vi "Control Lift.vi"(0 "Loop Time (ms)":u32=10, 2 "Lift Min Speed to Raise at (%)":dbl=-0.35, 5 "Lift Up PID Terms":cluster{"Kp":dbl, "Ki":dbl, "Kd":dbl}={"Kp"=0.1, "Ki"=0.0, "Kd"=0.0}) -> (14 "PID Tracking Lift Up":T1(graph)={"Goal"=0.0, "Process Variable"=-0.0345825, "Max Ouput"=0.0034582500000000004, 0.0345825, 0.0034582500000000004, 0.0, -0.0}, 15 "Current Error Lift":dbl=0.0345825)   [LabVIEW 2017]
uses:
  <vilib>/Rock Robotics/WPI/ThirdParty/Phoenix-LabVIEW/Motor Controller/Controls/CTRE_Phoenix_MotorControl_ControlMode.ctl
  <vilib>/Rock Robotics/WPI/DriverStation/WPI_DriverStationRobotMode2.ctl
  Globals/Robot Global Data.vi
  Globals/Manipulator Controller Inputs.vi
panel:
  in  "Lift Down Fast":bool=TRUE
  in  "Testing":bool
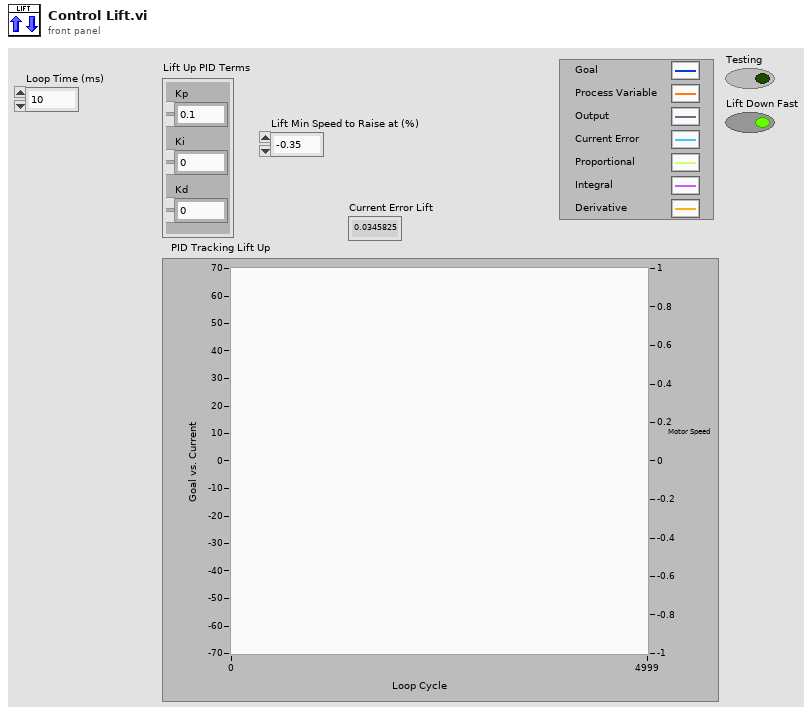
[diagram p1: front panel]
types:
  T1 = cluster{"Goal":dbl, "Process Variable":dbl, "Max Ouput":dbl, dbl, dbl, dbl, dbl}
  T2 = typedef "WPI_DriverStationRobotMode2.ctl" = enum16{"Autonomous Disabled", "Autonomous Enabled", "Teleop Disabled", "Teleop Enabled", "Disconnected", "Finish", "Test Disabled", "Test Enabled", "Emergency Stopped"}
  T3 = typedef "WPI_MotorControlDeviceRef.ctl" = cluster{"DeviceStatus":errorcluster, "Type":T4, "PWM":cluster{"PWM Channel":T5, "DeadBand":T6}, "CAN":cluster{"Device Number":u8, "SetOutput VI Ref":variant, "GetOutput VI Ref":variant, "Enable VI Ref":variant, "Disable VI Ref":variant, "Data":variant}, "Invert":bool, "DIO PWM":cluster{"PWM \"Enable\" Channel":T5, "DIOChannel":T7, "PWM Rate":dbl}}
  T4 = typedef "WPI_MotorControlType.ctl" = enum16{"PWM", "CAN", "DIO PWM"}
  T5 = typedef "FPGA_DIOPWMChannel.ctl" = enum8{"PWM 0", "PWM 1", "PWM 2", "PWM 3", "PWM 4", "PWM 5", "PWM 6", "PWM 7", "PWM 8", "PWM 9", "PWM MXP 0", "PWM MXP 1", "PWM MXP 2", "PWM MXP 3", "PWM MXP 4", "PWM MXP 5", "PWM MXP 6", "PWM MXP 7", "PWM MXP 8", "PWM MXP 9", "Invalid"}
  T6 = typedef "WPI_PWMDeadband.ctl" = cluster{"Name":string, "maxPositivePwm":i32, "minPositivePwm":i32, "centerPwm":i32, "maxNegativePwm":i32, "minNegativePwm":i32, "angularRange":u16}
  T7 = typedef "FPGA_DIOChannel.ctl" = enum8{"DIO 0", "DIO 1", "DIO 2", "DIO 3", "DIO 4", "DIO 5", "DIO 6", "DIO 7", "DIO 8", "DIO 9", "DIO MXP 0", "DIO MXP 1", "DIO MXP 2", "DIO MXP 3", "DIO MXP 4", "DIO MXP 5", "DIO MXP 6", "DIO MXP 7", "DIO MXP 8", "DIO MXP 9", "DIO MXP 10", "DIO MXP 11", "DIO MXP 12", "DIO MXP 13", "DIO MXP 14", "DIO MXP 15", "SPI Port CS1", "SPI Port CS2", "SPI Port CS3", "SPI Port MISO", "SPI Port MOSI", "Invalid"}
  T8 = typedef "CTRE_Phoenix_MotorControl_ControlMode.ctl" = u16
  T9 = typedef "WPI_DriverStationMatch Info.ctl" = cluster{"Autonomous Elapsed Seconds":dbl, "TeleOp Elapsed Seconds":dbl, "Disabled Elapsed Seconds":dbl, "Visited Autonomous":bool, "Visited TeleOp":bool, "Visited Disabled":bool, "Autonomous Settings":cluster{"Autonomous Style":enum16{"Iterative", "Independent"}, "VI Refnum":refnum<vi>}}
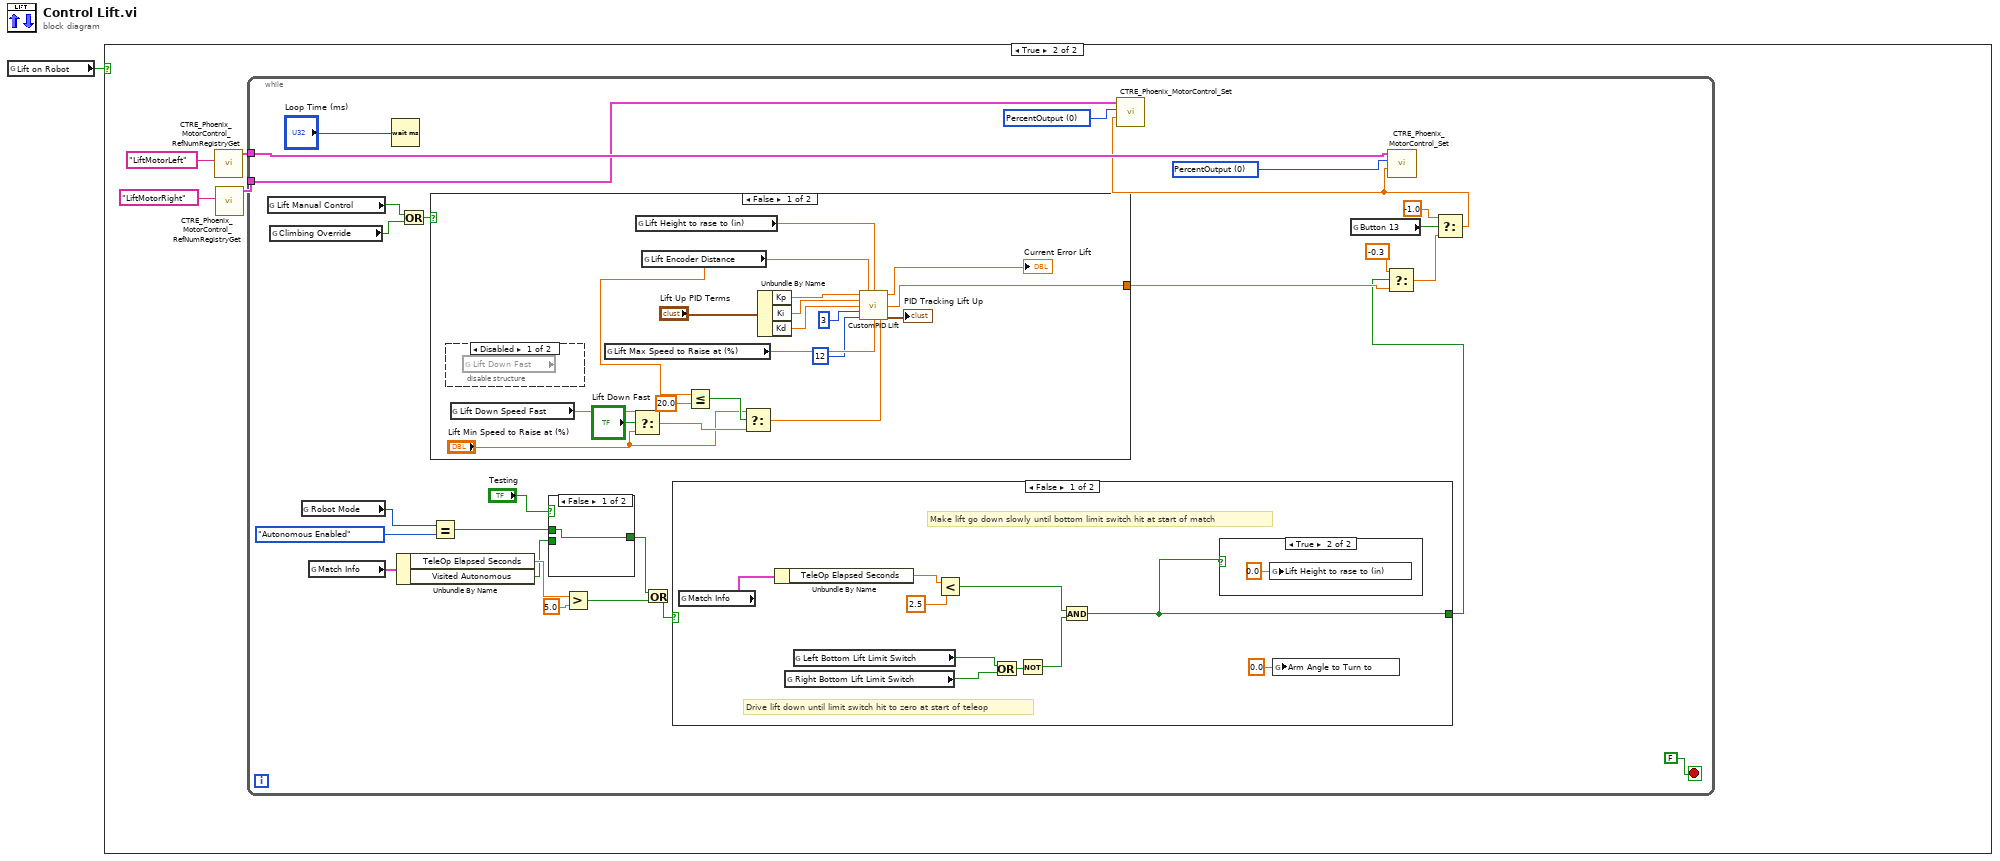
[diagram p0: block diagram]
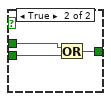
[diagram p3: hidden frame]
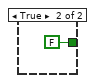
[diagram p5: hidden frame]
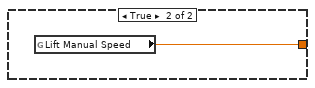
[diagram p7: hidden frame]
diagram:
  n1 = global read "Robot Global Data.vi" "Lift on Robot"() -> (w1:bool)
  n2 = case shown="True" w1 {
    frame False {
    }
    frame True {
      n3 = call "CTRE_Phoenix_MotorControl_RefNumRegistryGet.vi"("refnum name"="LiftMotorLeft") -> ("PhoenixMotorControlDevRef"=w5:T3)  [unwired: 9 in, 1 out]
      n4 = call "CTRE_Phoenix_MotorControl_RefNumRegistryGet.vi"("refnum name"="LiftMotorRight") -> ("PhoenixMotorControlDevRef"=w2:T3)  [unwired: 9 in, 1 out]
      n5 = while {
        tunnel: w5 -> [w31]
        tunnel: w2 -> [w27]
        stop <- FALSE stop-if-true
        w28 = T8 0 items=["PercentOutput"=0, "Position"=1, "Velocity"=2, "Current"=3, "Follower"=5, "MotionProfile"=6, "MotionMagic"=7, "MotionMagicArc"=8, "MotionProfileArc"=10, "Disabled"=15] ("Control Mode")
        w30 = T8 0 items=["PercentOutput"=0, "Position"=1, "Velocity"=2, "Current"=3, "Follower"=5, "MotionProfile"=6, "MotionMagic"=7, "MotionMagicArc"=8, "MotionProfileArc"=10, "Disabled"=15] ("Control Mode")
        n6 = global read "Robot Global Data.vi" "Lift Manual Control"() -> (w20:bool)
        n7 = global read "Robot Global Data.vi" "Climbing Override"() -> (w19:bool)
        n8 = global read "Robot Global Data.vi" "Robot Mode"() -> (w22:T2)
        n9 = global read "Robot Global Data.vi" "Match Info"() -> (w18:T9)
        n10 = Wait (ms)(milliseconds to wait="Loop Time (ms)") -> ()  [unwired: 1 out]
        n11 = Unbundle By Name(w18) -> ("TeleOp Elapsed Seconds"=w17:dbl, "Visited Autonomous"=w7:bool)
        n12 = Or(x=w20, y=w19) -> (x .or. y?=w21:bool)
        n13 = case shown="False" w21 {
          tunnel: [w67 w68] -> w26
          frame False {
            n14 = disable-structure shown="Disabled" {
              frame Disabled {
                n15 = global read "Robot Global Data.vi" "Lift Down Fast"() -> ()  [unwired: 1 out]
              }
              frame Enabled {
              }
            }
            n16 = global read "Robot Global Data.vi" "Lift Down Speed Fast"() -> (w56:dbl)
            n17 = global read "Robot Global Data.vi" "Lift Max Speed to Raise at (%)"() -> (w64:dbl)
            n18 = Select(t=w56, s="Lift Down Fast", f="Lift Min Speed to Raise at (%)") -> (s? t:f=w52:dbl)
            n19 = global read "Robot Global Data.vi" "Lift Height to rase to (in)"() -> (w65:dbl)
            n20 = global read "Robot Global Data.vi" "Lift Encoder Distance"() -> (w55:dbl)
            n21 = Less Or Equal?(x=w55, y=20.0) -> (x <= y?=w53:bool)
            n22 = Select(t="Lift Min Speed to Raise at (%)", s=w53, f=w52) -> (s? t:f=w50:dbl)
            n23 = Unbundle By Name("Lift Up PID Terms") -> ("Kp"=w59:dbl, "Ki"=w58:dbl, "Kd"=w57:dbl)
            n24 = call "CustomPID Lift.vi"("Kp"=w59, "Process Variable"=w55, "Goal"=w65, "Ki"=w58, "Kd"=w57, "N-Diff"=3, "N-Int"=12, "Max Ouput"=w64, "Min Output"=w50) -> ("Current Error"=→"Current Error Lift":dbl, "Command"=w67:dbl, "PID Tracking"=→"PID Tracking Lift Up":T1)  [unwired: 4 in]
          }
          frame True {
            n25 = global read "Robot Global Data.vi" "Lift Manual Speed"() -> (w68:dbl)
          }
        }
        n26 = Equal?(x=w22, y=WPI_DriverStationRobotMode2."Autonomous Enabled" ("Robot Mode")) -> (x = y?=w8:bool)
        n27 = case shown="False" "Testing" {
          tunnel: [w33 w36] -> w9
          tunnel: w8 -> [w33 w35]
          tunnel: w7 -> [_ w34]
          frame False {
          }
          frame True {
            n28 = Or(x=w35, y=w34) -> (x .or. y?=w36:bool)
          }
        }
        n29 = Greater?(x=w17, y=5.0) -> (0:w15:bool)
        n30 = Or(x=w9, y=w15) -> (x .or. y?=w10:bool)
        n31 = case shown="False" w10 {
          tunnel: [w38 FALSE] -> w24
          frame False {
            # "Drive lift down until limit switch hit to zero at start of teleop"
            # "Make lift go down slowly until bottom limit switch hit at start of match"
            n32 = global read "Robot Global Data.vi" "Match Info"() -> (w46:T9)
            n33 = Unbundle By Name(w46) -> ("TeleOp Elapsed Seconds"=w39:dbl)
            n34 = global read "Robot Global Data.vi" "Right Bottom Lift Limit Switch"() -> (w43:bool)
            n35 = global read "Robot Global Data.vi" "Left Bottom Lift Limit Switch"() -> (w44:bool)
            n36 = Less?(x=w39, y=2.5) -> (x < y?=w40:bool)
            n37 = Or(x=w44, y=w43) -> (x .or. y?=w42:bool)
            n38 = Not(x=w42) -> (.not. x?=w41:bool)
            n39 = And(x=w40, y=w41) -> (x .and. y?=w38:bool)
            n40 = case shown="True" w38 {
              frame False {
              }
              frame True {
                n41 = global write "Robot Global Data.vi" "Lift Height to rase to (in)"(0.0 ("Lift Height to rase to (in)")) -> ()
              }
            }
            n42 = global write "Robot Global Data.vi" "Arm Angle to Turn to"(0.0 ("Arm Angle to Turn to")) -> ()
          }
          frame True {
          }
        }
        n43 = global read "Manipulator Controller Inputs.vi" "Button 13"() -> (w14:bool)
        n44 = Select(t=-0.3, s=w24, f=w26) -> (s? t:f=w13:dbl)
        n45 = Select(t=-1.0, s=w14, f=w13) -> (s? t:f=w12:dbl)
        n46 = call <vilib>:"CTRE_Phoenix_MotorControl_Set.vi"("Output"=w12, "Control Mode"=w28, "PhoenixMotorControlDevRef"=w27) -> ()  [unwired: 7 in, 2 out]
        n47 = call <vilib>:"CTRE_Phoenix_MotorControl_Set.vi"("Output"=w12, "Control Mode"=w30, "PhoenixMotorControlDevRef"=w31) -> ()  [unwired: 7 in, 2 out]
      }
    }
  }
